vi "Commence Analog Output Null Measurement.vi"(8 "error in (no error)":errorcluster, 11 "VISA resource name":refnum<visa-resource-name>) -> (0 "error out":errorcluster, 3 "VISA resource name out":refnum<visa-resource-name>)   [LabVIEW 2021, in "Agilent 34420.lvlib"]
doc: "Sets the next measurement to a null measurement for the analog out port (on the back of the instrument).\n\nAnalog out port basically scales the readings taken at the measurement port and allows the user to keep track of or to graph the measurements. However a much better and easier way to do this would be taking the measurements using the <B>Read (Multiple Points)</B> or <B>Initiate</B> & <B>Fetch Multiple Points</B> VIs and then graphing the acquired data programmatically.\n\n<B>Note:</B>\n\nThe test equipment (leads, loads, etc.) that will be nulled should be connected to the front of the instrument before the measurement is taken."
uses:
  <instrlib>/Agilent 34420/Agilent 34420.lvlib
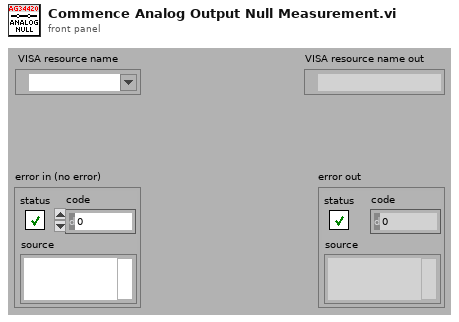
[diagram p1: front panel]
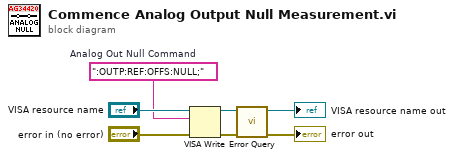
[diagram p0: block diagram]
diagram:
  w1 = ":OUTP:REF:OFFS:NULL;"  # Analog Out Null Command
  n1 = VISA Write(VISA resource name="VISA resource name", write buffer=w1, error in (no error)="error in (no error)") -> (VISA resource name out=w3:refnum<visa-resource-name>, error out=w2:errorcluster)  [unwired: 1 out]
  n2 = call <instrlib>:"Error Query.vi"("error in (no error)"=w2, "VISA resource name"=w3) -> ("error out"=→"error out":errorcluster, "VISA resource name out"=→"VISA resource name out":refnum<visa-resource-name>)  [unwired: 6 in, 2 out]
